vi "PH_HamamatsuCamera.PC Cam Parameter.vi"(0 "VI in":refnum<vi>, 1 "Parameter Name":string, 2 "Wanted Value":dbl, 5 "error in (no error)":errorcluster) -> (14 "VI out":refnum<vi>, 19 "error out":errorcluster)   [LabVIEW 2014, in "PH_HamamatsuCamera.lvlib"]
uses:
  PH_HamamatsuCamera.lvlib
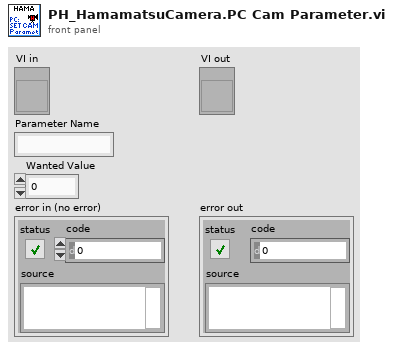
[diagram p1: front panel]
types:
  T1 = typedef "PH_HamamatsuCamera.lvlib/PH_HamamatsuCamera.i attribute.ctl" = cluster{"Gui Refs":cluster{"Camera Details":refnum<vi>, "ROI":refnum<vi>, "Set ROI to Maximum":refnum<vi>, "Trigger Parameters":refnum<vi>, "Brightness":refnum<vi>, "Shutter":refnum<vi>, "Gain":refnum<vi>, "Trigger Timeout":refnum<vi>, "Trigger Polarity":refnum<vi>, "Trigger Mode":refnum<vi>, "Parameters":refnum<vi>, "Set Cam Parameter":refnum<vi>, "Parameter to set":refnum<vi>, "Value to set":refnum<vi>}, "Cam":cluster{"Handle":i32, "Details":cluster{"Model":string, "Camera ID":string, "Firmware":string}, "Buffer Info":cluster{"height":u32, "width":u32, "datatype":u32}}, "H Offset":cluster{"Value":i32, "Minimum":i32, "Maximum":i32, "Increment":i32}, "V Offset":cluster{"Value":i32, "Minimum":i32, "Maximum":i32, "Increment":i32}, "H Width":cluster{"Value":i32, "Minimum":i32, "Maximum":i32, "Increment":i32}, "V Width":cluster{"Value":i32, "Minimum":i32, "Maximum":i32, "Increment":i32}, "Trigger Parameters":T2, "Trigger Timeout":u32, "Parameters":T3[], "Indicees Cam Parameters":cluster{"Brightness":i32, "Shutter":i32, "Gain":i32}, "Wanted Values":cluster{"Trigger Settings":T2[], "ROI":T4[], "Parameter":cluster{"Name":string, "Value":dbl}[]}}
  T2 = typedef "PH_HamamatsuCamera.lvlib/PH_HamamatsuCamera.Trigger Parameter.ctl" = cluster{"Mode":u32, "Polarity":u32, "Times":u32, "Delay":dbl}
  T3 = typedef "PH_HamamatsuCamera.lvlib/PH_HamamatsuCamera.Parameter Set.ctl" = cluster{"Parameter":string, "Value":dbl, "Writable":bool, "Range":cluster{"min":dbl, "max":dbl, "step":dbl}, "Default":dbl, "Value Names":cluster{"Name":string, "Value":dbl}[], "Text Values":bool}
  T4 = typedef "PH_HamamatsuCamera.lvlib/PH_HamamatsuCamera.ROI.ctl" = cluster{"Horizontal Offset":i32, "Vertical Offset":i32, "Horizontal Width":i32, "Vertical Width":i32}
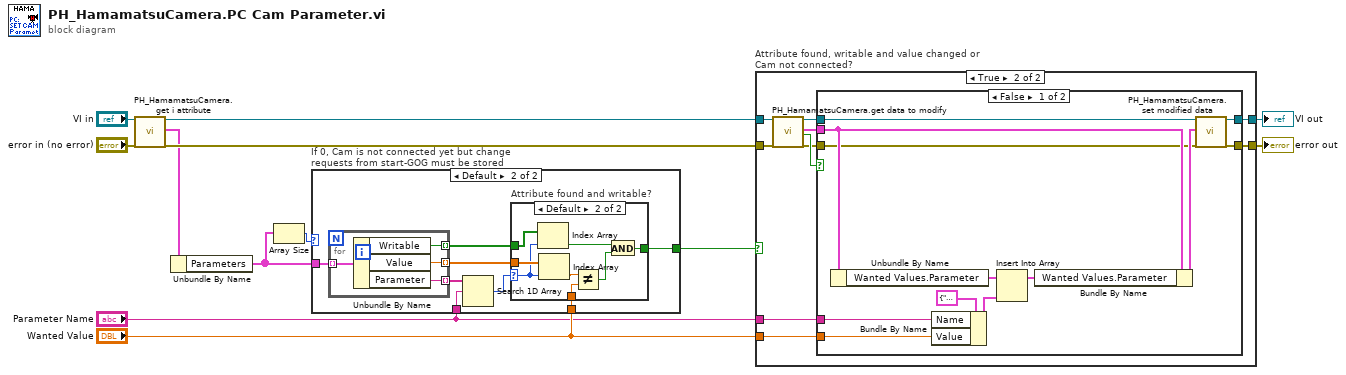
[diagram p0: block diagram]
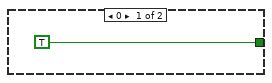
[diagram p2: hidden frame]
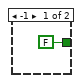
[diagram p3: hidden frame]
diagram:
  n1 = call "PH_HamamatsuCamera.get i attribute.vi"("i ref in"="VI in", "error in (no error)"="error in (no error)") -> ("i ref out"=w9:refnum<vi>, "i attribute"=w8:T1, "error out"=w11:errorcluster)  [unwired: 15 in]
  n2 = Unbundle By Name(w8) -> ("Parameters"=w2:T3[])
  n3 = Array Size(array=w2) -> (size(s)=w1:i32)
  n4 = case "If 0, Cam is not connected yet but change requests from start-GOG must be stored" shown="Default" w1 {
    tunnel: "Wanted Value" -> [_ w21]
    tunnel: w2 -> [_ w19]
    tunnel: [TRUE w16] -> w4
    tunnel: "Parameter Name" -> [_ w15]
    frame 0 {
    }
    frame Default {
      n5 = for {
        tunnel: w19 -> [w34] mode=indexing
        tunnel: [w33] -> w20 mode=indexing
        tunnel: [w32] -> w18 mode=indexing
        tunnel: [w31] -> w17 mode=indexing
        n6 = Unbundle By Name(w34) -> ("Writable"=w31:bool, "Value"=w32:dbl, "Parameter"=w33:string)
      }
      n7 = Search 1D Array(1D array=w20, element=w15) -> (index of element=w14:i32)  [unwired: 1 in]
      n8 = case "Attribute found and writable?" shown="Default" w14 {
        selector: w14 -> [_ w23]
        tunnel: w21 -> [_ w30]
        tunnel: w18 -> [_ w29]
        tunnel: w17 -> [_ w28]
        tunnel: [FALSE w24] -> w16
        frame -1 {
        }
        frame Default {
          n9 = Index Array(array=w28, index=w23) -> (element=w26:bool)
          n10 = Index Array(array=w29, index=w23) -> (element=w27:dbl)
          n11 = Not Equal?(x=w27, y=w30) -> (x != y?=w25:bool)
          n12 = And(x=w26, y=w25) -> (x .and. y?=w24:bool)
        }
      }
    }
  }
  n13 = case "Attribute found, writable and value changed or Cam not connected?" shown="True" w4 {
    tunnel: [w35 w44] -> w12
    tunnel: w11 -> [w35 w43]
    tunnel: [w36 w42] -> w10
    tunnel: w9 -> [w36 w41]
    tunnel: "Wanted Value" -> [_ w38]
    tunnel: "Parameter Name" -> [_ w37]
    frame False {
    }
    frame True {
      n14 = call "PH_HamamatsuCamera.get data to modify.vi"("i ref in"=w41, "error in (no error)"=w43) -> ("i ref out"=w39:refnum<vi>, "i attribute"=w46:T1, "timed out"=w45:bool, "error out"=w40:errorcluster)  [unwired: 14 in]
      n15 = case shown="False" w45 {
        tunnel: w39 -> [w58 w60]
        tunnel: w40 -> [w51 w59]
        tunnel: [w53 w60] -> w42
        tunnel: [w52 w59] -> w44
        tunnel: w46 -> [w56 _]
        tunnel: w38 -> [w48 _]
        tunnel: w37 -> [w47 _]
        frame False {
          n16 = Unbundle By Name(w56) -> ("Wanted Values.Parameter"=w55:cluster{"Name":string, "Value":dbl}[])
          n17 = Bundle By Name(cluster=cluster{"Name":string, "Value":dbl} {"Name"="", "Value"=0.0} ("new element/subarray"), "Name"=w47, "Value"=w48) -> (w49:cluster{"Name":string, "Value":dbl})
          n18 = Insert Into Array(array=w55, new element=w49) -> (w54:cluster{"Name":string, "Value":dbl}[])  [unwired: 1 in]
          n19 = Bundle By Name(cluster=w56, "Wanted Values.Parameter"=w54) -> (w57:T1)
          n20 = call "PH_HamamatsuCamera.set modified data.vi"("i ref in"=w58, "i attribute"=w57, "error in (no error)"=w51) -> ("i ref out"=w53:refnum<vi>, "error out"=w52:errorcluster)  [unwired: 15 in]
        }
        frame True {
        }
      }
    }
  }
  "error out" <- w12
  "VI out" <- w10
